vi "类型2自动测试.vi"() -> ()   [LabVIEW 2010]
uses:
  全局量/试验配置信息.vi
panel:
  in  "数组_选择":bool[](array[boolean])
  in  "记录跳变次数":i32
  in  "变化量":dbl
  in  "当前波动值":dbl
  in  "最近一次跳变防线值":i32
  in  "发送值状态":i32
  in  "反馈值":i32
  in  "发送值":dbl
  out "合格？":bool[][](array[boolean])
  in  "跳变值 2":dbl[](array[numeric])
  in  "跳变值 1":dbl[](array[numeric])
  in  "误差":dbl[][](array[numeric])
  out "EVENT_KEY":string
  out "bRece":bool
  out "bSend":bool
  out "bStop":bool
  out "第几组":i32
  # "SEND_RISE = 1,//递增\n\tSEND_SUB = 2,//递减\n\tSEND_OVER = 3//发送完毕"
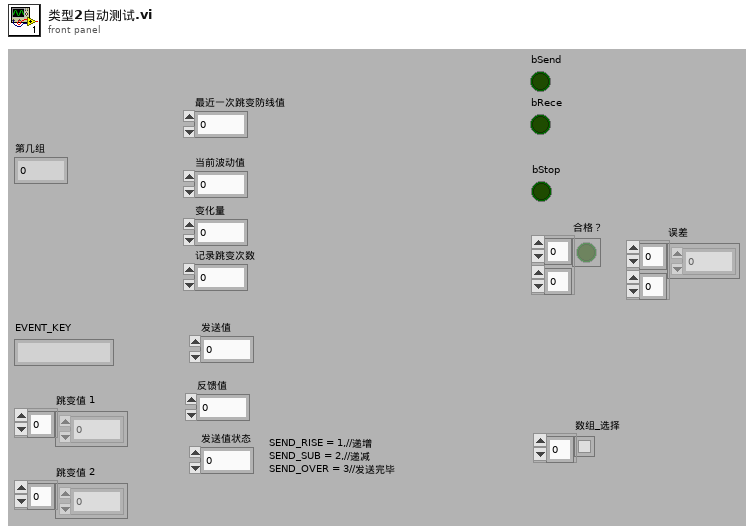
[diagram p1: front panel]
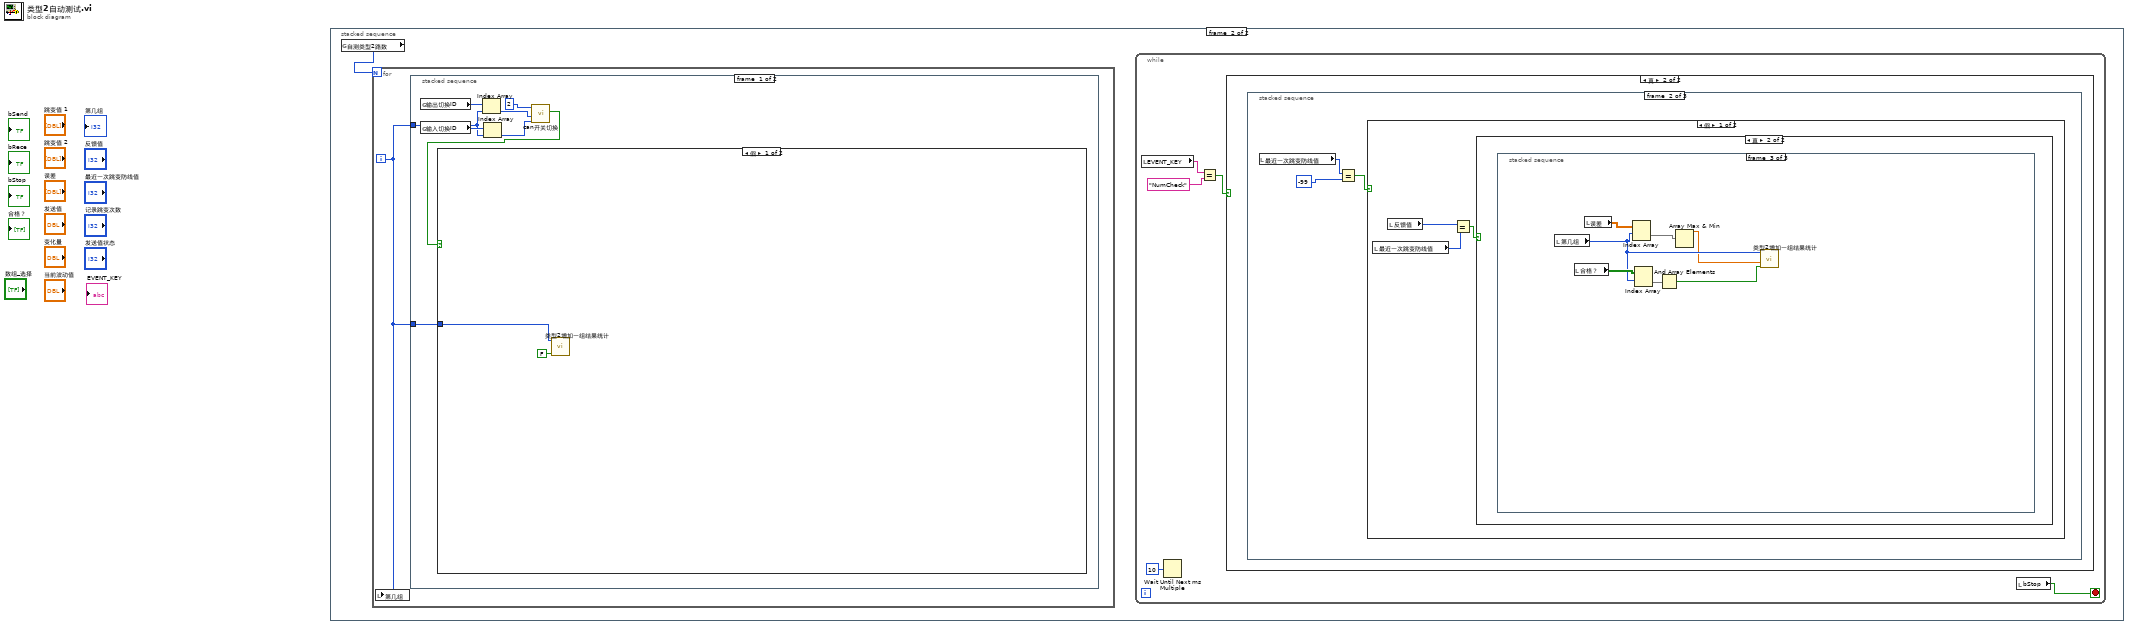
[diagram p0: block diagram]
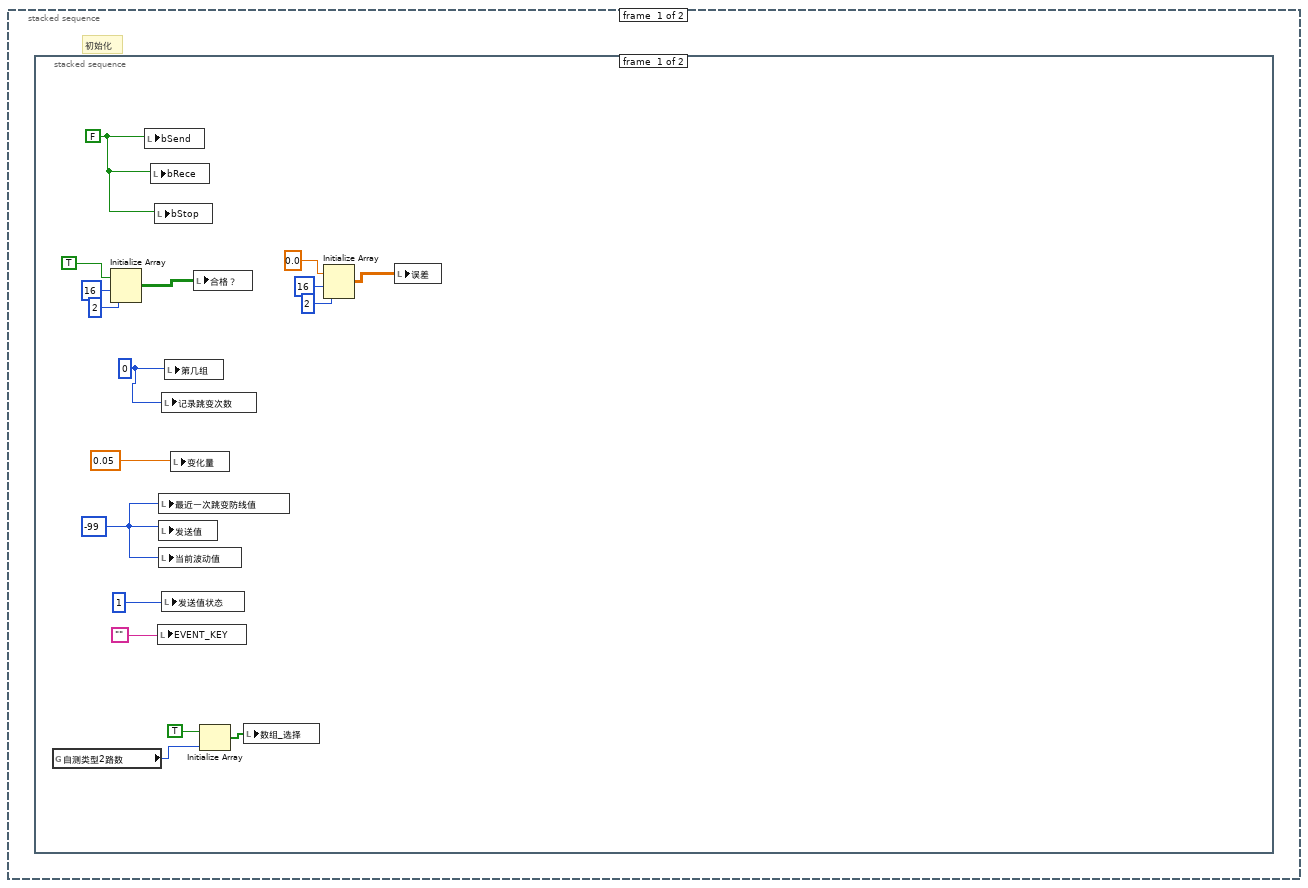
[diagram p2: hidden frame]
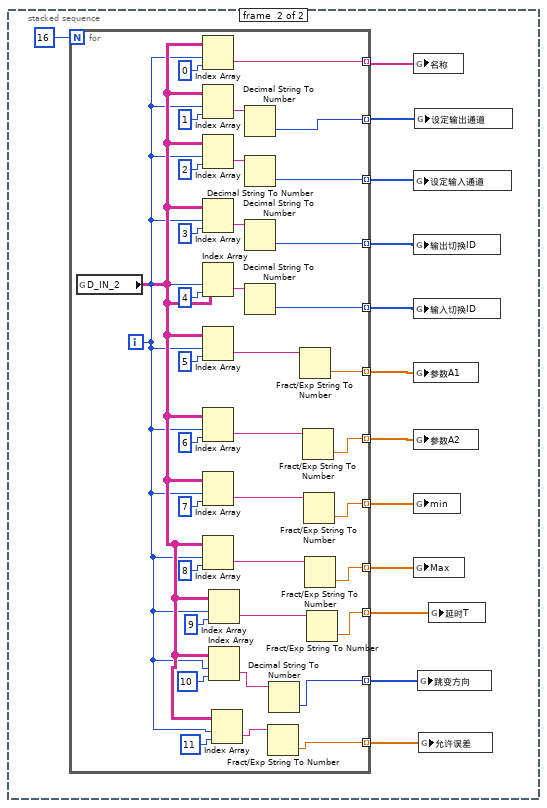
[diagram p3: hidden frame]
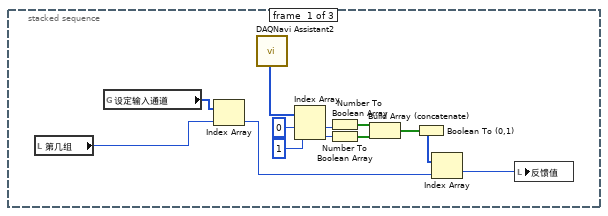
[diagram p5: hidden frame]
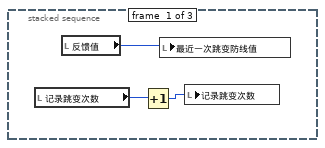
[diagram p7: hidden frame]
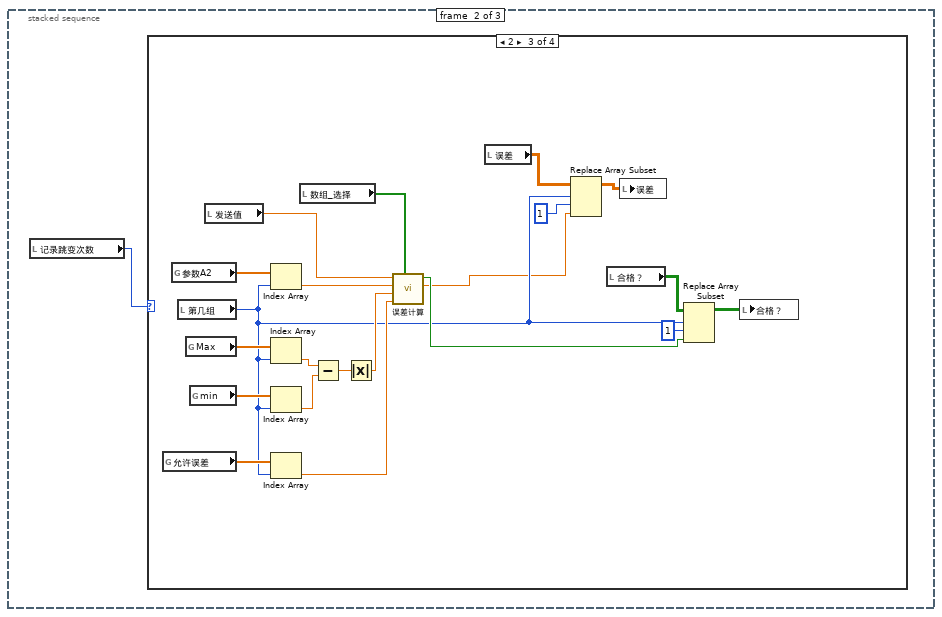
[diagram p8: hidden frame]
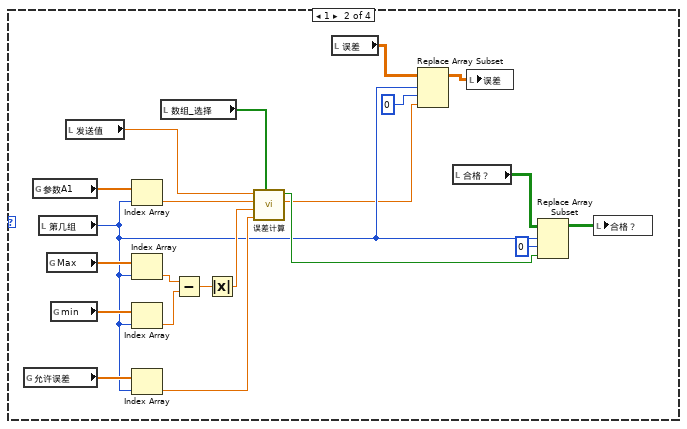
[diagram p10: hidden frame]
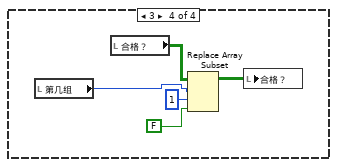
[diagram p11: hidden frame]
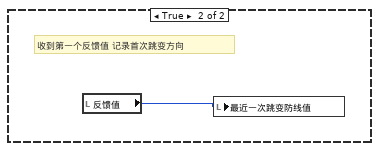
[diagram p12: hidden frame]
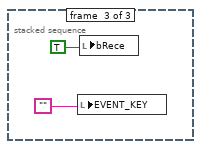
[diagram p13: hidden frame]
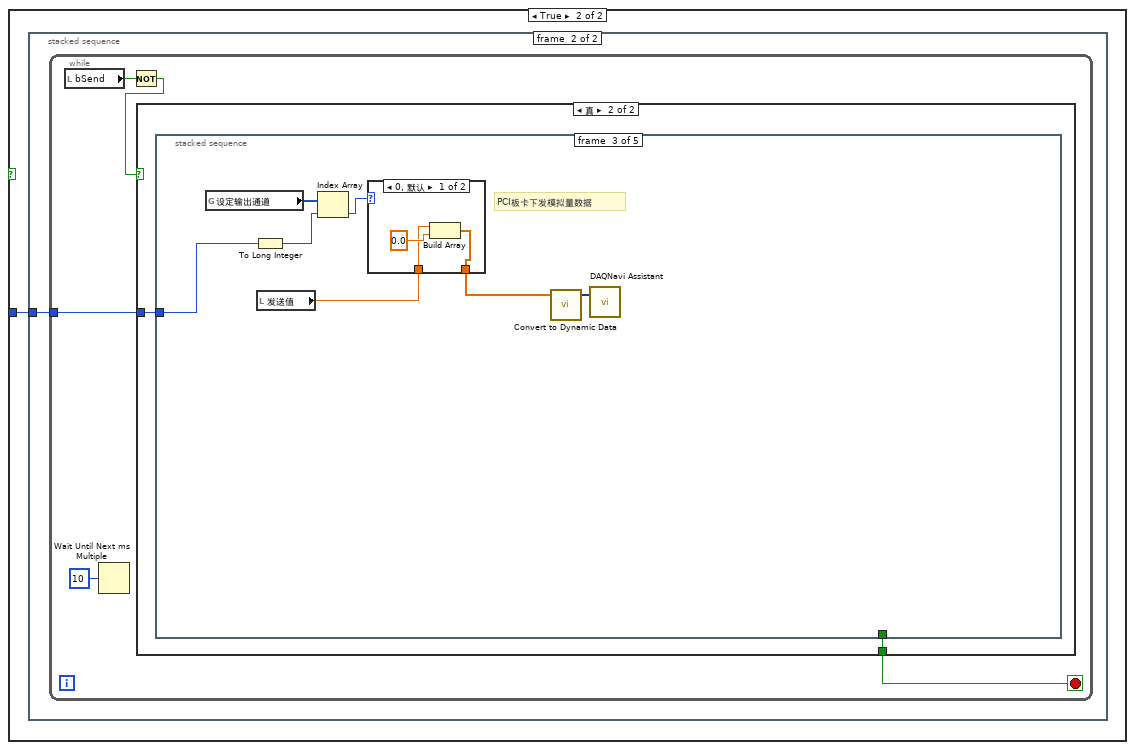
[diagram p14: hidden frame]
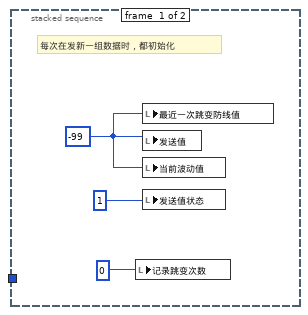
[diagram p15: hidden frame]
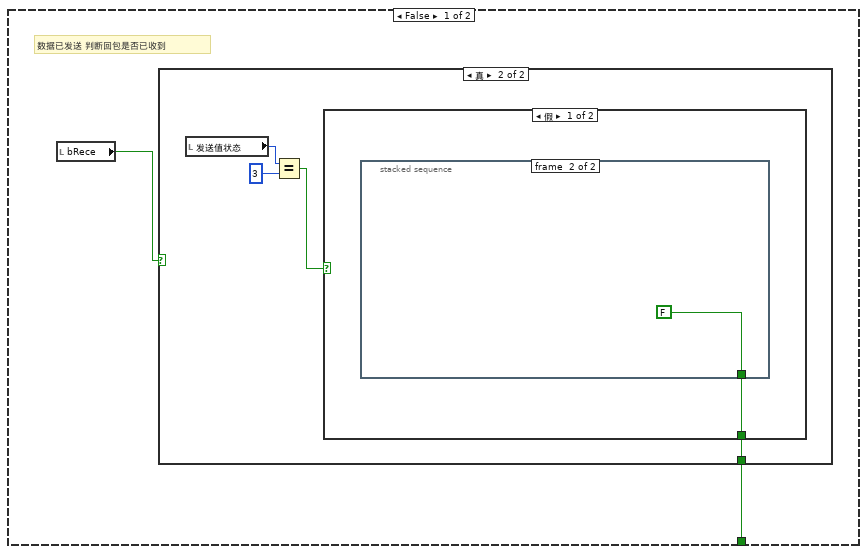
[diagram p16: hidden frame]
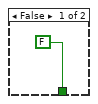
[diagram p17: hidden frame]
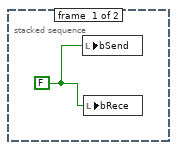
[diagram p18: hidden frame]
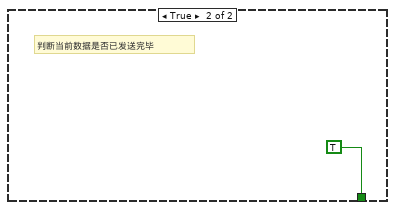
[diagram p19: hidden frame]
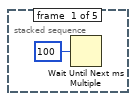
[diagram p20: hidden frame]
diagram:
  n1 = stacked-sequence {
    frame #0 {
      # "初始化"
      n2 = stacked-sequence {
        frame #0 {
          w10 = -99
          w11 = 0
          w17 = FALSE
          n3 = global read "试验配置信息.vi" "自测类型2路数"() -> (w5:i32)
          n4 = Initialize Array(TRUE, 16 ("维数大小"), 2 ("维数大小")) -> (w14:bool[][])
          n5 = local write "bSend"(w17) -> ()
          n6 = local write "bRece"(w17) -> ()
          n7 = local write "bStop"(w17) -> ()
          n8 = local write "EVENT_KEY"("") -> ()
          n9 = local write "最近一次跳变防线值"(w10) -> ()
          n10 = local write "发送值"(w10) -> ()
          n11 = local write "当前波动值"(w10) -> ()
          n12 = local write "记录跳变次数"(w11) -> ()
          n13 = local write "发送值状态"(1) -> ()
          n14 = local write "第几组"(w11) -> ()
          n15 = local write "变化量"(0.05) -> ()
          n16 = local write "合格？"(w14) -> ()
          n17 = Initialize Array(TRUE, w5) -> (w7:bool[])
          n18 = local write "数组_选择"(w7) -> ()
          n19 = Initialize Array(0.0, 16 ("维数大小"), 2 ("维数大小")) -> (w2:dbl[][])
          n20 = local write "误差"(w2) -> ()
        }
        frame #1 {
          n21 = for {
            N: 16 ("维数大小") -> [_]
            tunnel: [w66] -> w24 mode=indexing
            tunnel: [w62] -> w23 mode=indexing
            tunnel: [w60] -> w22 mode=indexing
            tunnel: [w57] -> w21 mode=indexing
            tunnel: [w54] -> w20 mode=indexing
            tunnel: [w51] -> w26 mode=indexing
            tunnel: [w48] -> w27 mode=indexing
            tunnel: [w45] -> w28 mode=indexing
            tunnel: [w42] -> w29 mode=indexing
            tunnel: [w39] -> w30 mode=indexing
            tunnel: [w32] -> w19 mode=indexing
            tunnel: [w31] -> w18 mode=indexing
            i -> [w33]
            n22 = global read "试验配置信息.vi" "D_IN_2"() -> (w34:string[][])
            n23 = Index Array(array=w34, index (row)=w33, index (col)=0 ("禁用的索引 (列)")) -> (element=w66:string)
            n24 = Index Array(array=w34, index (row)=w33, index (col)=1 ("禁用的索引 (列)")) -> (element=w59:string)
            n25 = Index Array(array=w34, index (row)=w33, index (col)=2 ("禁用的索引 (列)")) -> (element=w56:string)
            n26 = Index Array(array=w34, index (row)=w33, index (col)=3 ("禁用的索引 (列)")) -> (element=w52:string)
            n27 = Index Array(array=w34, index (row)=w33, index (col)=4 ("禁用的索引 (列)")) -> (element=w50:string)
            n28 = Index Array(array=w34, index (row)=w33, index (col)=5 ("禁用的索引 (列)")) -> (element=w47:string)
            n29 = Index Array(array=w34, index (row)=w33, index (col)=6 ("禁用的索引 (列)")) -> (element=w43:string)
            n30 = Index Array(array=w34, index (row)=w33, index (col)=7 ("禁用的索引 (列)")) -> (element=w63:string)
            n31 = Index Array(array=w34, index (row)=w33, index (col)=8 ("禁用的索引 (列)")) -> (element=w61:string)
            n32 = Index Array(array=w34, index (row)=w33, index (col)=9 ("禁用的索引 (列)")) -> (element=w40:string)
            n33 = Index Array(array=w34, index (row)=w33, index (col)=10 ("禁用的索引 (列)")) -> (element=w35:string)
            n34 = Index Array(array=w34, index (row)=w33, index (col)=11 ("禁用的索引 (列)")) -> (element=w36:string)
            n35 = Decimal String To Number(string=w59) -> (number=w57:i32)  [unwired: 2 in, 1 out]
            n36 = Decimal String To Number(string=w56) -> (number=w54:i32)  [unwired: 2 in, 1 out]
            n37 = Decimal String To Number(string=w52) -> (number=w51:i32)  [unwired: 2 in, 1 out]
            n38 = Decimal String To Number(string=w50) -> (number=w48:i32)  [unwired: 2 in, 1 out]
            n39 = Fract/Exp String To Number(string=w36) -> (number=w31:dbl)  [unwired: 3 in, 1 out]
            n40 = Decimal String To Number(string=w35) -> (number=w32:i32)  [unwired: 2 in, 1 out]
            n41 = Fract/Exp String To Number(string=w47) -> (number=w45:dbl)  [unwired: 3 in, 1 out]
            n42 = Fract/Exp String To Number(string=w43) -> (number=w42:dbl)  [unwired: 3 in, 1 out]
            n43 = Fract/Exp String To Number(string=w63) -> (number=w62:dbl)  [unwired: 3 in, 1 out]
            n44 = Fract/Exp String To Number(string=w61) -> (number=w60:dbl)  [unwired: 3 in, 1 out]
            n45 = Fract/Exp String To Number(string=w40) -> (number=w39:dbl)  [unwired: 3 in, 1 out]
          }
          n46 = global write "试验配置信息.vi" "名称"(w24) -> ()
          n47 = global write "试验配置信息.vi" "设定输入通道"(w20) -> ()
          n48 = global write "试验配置信息.vi" "输出切换ID"(w26) -> ()
          n49 = global write "试验配置信息.vi" "输入切换ID"(w27) -> ()
          n50 = global write "试验配置信息.vi" "参数A1"(w28) -> ()
          n51 = global write "试验配置信息.vi" "参数A2"(w29) -> ()
          n52 = global write "试验配置信息.vi" "min"(w23) -> ()
          n53 = global write "试验配置信息.vi" "Max"(w22) -> ()
          n54 = global write "试验配置信息.vi" "设定输出通道"(w21) -> ()
          n55 = global write "试验配置信息.vi" "跳变方向"(w19) -> ()
          n56 = global write "试验配置信息.vi" "允许误差"(w18) -> ()
          n57 = global write "试验配置信息.vi" "延时T"(w30) -> ()
        }
      }
    }
    frame #1 {
      n58 = global read "试验配置信息.vi" "自测类型2路数"() -> (w68:i32)
      n59 = for {
        N: w68 -> [_]
        i -> [w154]
        n60 = local write "第几组"(w154) -> ()
        n61 = stacked-sequence {
          tunnel: w154 -> [w157 _]
          tunnel: w154 -> [w155 _]
          frame #0 {
            n62 = global read "试验配置信息.vi" "输出切换ID"() -> (w159:i32[])
            n63 = global read "试验配置信息.vi" "输入切换ID"() -> (w160:i32[])
            n64 = Index Array(array=w159, index=w157) -> (element=w158:i32)
            n65 = Index Array(array=w160, index=w157) -> (element=w161:i32)
            n66 = call "can开关切换.vi"("输入切换ID"=w161, "输出切换ID"=w158, "函数类型"=2) -> ("成功？"=w156:bool)  [unwired: 7 in]
            n67 = case shown="假" w156 {
              tunnel: w155 -> [w164 w165]
              frame False {
                n68 = call "类型2增加一组结果统计.vi"("合格"=FALSE, "第几组"=w164) -> ()  [unwired: 10 in]
              }
              frame True {
                n69 = stacked-sequence {
                  tunnel: w165 -> [_ w169]
                  frame #0 {
                    w168 = -99
                    # "每次在发新一组数据时，都初始化"
                    n70 = local write "记录跳变次数"(0) -> ()
                    n71 = local write "最近一次跳变防线值"(w168) -> ()
                    n72 = local write "发送值"(w168) -> ()
                    n73 = local write "当前波动值"(w168) -> ()
                    n74 = local write "发送值状态"(1) -> ()
                  }
                  frame #1 {
                    n75 = while {
                      tunnel: w169 -> [w172]
                      stop <- w171 stop-if-true
                      n76 = local read "bSend"() -> (w174:bool)
                      n77 = Wait Until Next ms Multiple(millisecond multiple=u32 10 ("毫秒倍数")) -> ()  [unwired: 1 out]
                      n78 = Not(x=w174) -> (.not. x?=w173:bool)
                      n79 = case shown="真" w173 {
                        tunnel: w172 -> [_ w187]
                        tunnel: [w175 w186] -> w171
                        frame False {
                          # "数据已发送 判断回包是否已收到"
                          n80 = local read "bRece"() -> (w176:bool)
                          n81 = case shown="真" w176 {
                            tunnel: [FALSE w178] -> w175
                            frame False {
                            }
                            frame True {
                              n82 = local read "发送值状态"() -> (w181:i32)
                              n83 = Equal?(x=w181, y=3) -> (x = y?=w179:bool)
                              n84 = case shown="假" w179 {
                                tunnel: [w182 TRUE] -> w178
                                frame False {
                                n85 = stacked-sequence {
                                tunnel: [_ FALSE] -> w182
                                frame #0 {
                                w183 = FALSE
                                n86 = local write "bSend"(w183) -> ()
                                n87 = local write "bRece"(w183) -> ()
                                }
                                frame #1 {
                                }
                                }
                                }
                                frame True {
                                # "判断当前数据是否已发送完毕"
                                }
                              }
                            }
                          }
                        }
                        frame True {
                          n88 = stacked-sequence {
                            tunnel: w187 -> [_ _ w216 _ _]
                            tunnel: [_ _ _ _ FALSE] -> w186
                            frame #0 {
                              n89 = Wait Until Next ms Multiple(millisecond multiple=u32 100 ("毫秒倍数")) -> ()  [unwired: 1 out]
                            }
                            frame #1 {
                              n90 = local read "发送值"() -> (w191:dbl)
                              n91 = Equal?(x=w191, y=-99.0) -> (x = y?=w189:bool)
                              n92 = case shown="假" w189 {
                                frame False {
                                n93 = local read "发送值状态"() -> (w192:i32)
                                n94 = case shown="1, 默认" w192 {
                                frame 1, Default {
                                # "当前状态是递增"
                                n95 = stacked-sequence {
                                frame #0 {
                                n96 = local read "发送值"() -> (w195:dbl)
                                n97 = local read "变化量"() -> (w194:dbl)
                                n98 = Add(x=w195, y=w194) -> (x+y=w193:dbl)
                                n99 = local write "发送值"(w193) -> ()
                                }
                                frame #1 {
                                n100 = local read "第几组"() -> (w199:i32)
                                n101 = global read "试验配置信息.vi" "Max"() -> (w200:dbl[])
                                n102 = local read "发送值"() -> (w198:dbl)
                                n103 = Index Array(array=w200, index=w199) -> (element=w196:dbl)
                                n104 = Greater Or Equal?(x=w198, y=w196) -> (x >= y?=w197:bool)
                                n105 = case shown="真" w197 {
                                tunnel: w196 -> [_ w202]
                                frame False {
                                }
                                frame True {
                                # "超过最大值时\n将状态改为递减状态"
                                n106 = local write "发送值"(w202) -> ()
                                n107 = local write "发送值状态"(2 ("发送值状态")) -> ()
                                }
                                }
                                }
                                }
                                }
                                frame 2 {
                                # "当前状态为递减状态"
                                n108 = stacked-sequence {
                                frame #0 {
                                n109 = local read "发送值"() -> (w205:dbl)
                                n110 = local read "变化量"() -> (w204:dbl)
                                n111 = Subtract(x=w205, y=w204) -> (x-y=w203:dbl)
                                n112 = local write "发送值"(w203) -> ()
                                }
                                frame #1 {
                                n113 = local read "第几组"() -> (w209:i32)
                                n114 = global read "试验配置信息.vi" "min"() -> (w210:dbl[])
                                n115 = local read "发送值"() -> (w208:dbl)
                                n116 = Index Array(array=w210, index=w209) -> (element=w206:dbl)
                                n117 = Less Or Equal?(x=w208, y=w206) -> (x <= y?=w207:bool)
                                n118 = case shown="真" w207 {
                                tunnel: w206 -> [_ w212]
                                frame False {
                                }
                                frame True {
                                # "递减到最小值时 代表发送了一个周期"
                                n119 = local write "发送值"(w212) -> ()
                                n120 = local write "发送值状态"(3 ("发送值状态")) -> ()
                                }
                                }
                                }
                                }
                                }
                                }
                                }
                                frame True {
                                # "默认值 证明为发送的第一条数据\n从最小值开始"
                                n121 = local read "第几组"() -> (w213:i32)
                                n122 = global read "试验配置信息.vi" "min"() -> (w215:dbl[])
                                n123 = Index Array(array=w215, index=w213) -> (element=w214:dbl)
                                n124 = local write "发送值"(w214) -> ()
                                }
                              }
                            }
                            frame #2 {
                              # "PCI板卡下发模拟量数据"
                              n125 = global read "试验配置信息.vi" "设定输出通道"() -> (w222:i32[])
                              n126 = To Long Integer(number=w216) -> (32bit integer=w221:i32)
                              n127 = local read "发送值"() -> (w217:dbl)
                              n128 = Index Array(array=w222, index=w221) -> (element=w218:i32)
                              n129 = case shown="0, 默认" w218 {
                                tunnel: [w225 w228] -> w219
                                tunnel: w217 -> [w223 w226]
                                frame 0, Default {
                                n130 = Build Array(w223, 0.0) -> (w225:dbl[])
                                }
                                frame 1 {
                                n131 = Build Array(0.0, w226) -> (w228:dbl[])
                                }
                              }
                              n132 = call "Convert to Dynamic Data"("Array"=w219) -> ("Dynamic Data Type"=w220:dynamicdata)  [unwired: 3 out]
                              n133 = call "DAQNavi Assistant"("data in(DDT)"=w220) -> ()  [unwired: 2 in, 17 out]
                            }
                            frame #3 {
                              n134 = local write "EVENT_KEY"("NumCheck") -> ()
                            }
                            frame #4 {
                              n135 = local write "bSend"(TRUE) -> ()
                            }
                          }
                        }
                      }
                    }
                  }
                }
              }
            }
          }
          frame #1 {
            n136 = local read "第几组"() -> (w233:i32)
            n137 = global read "试验配置信息.vi" "自测类型2路数"() -> (w235:i32)
            n138 = Decrement(x=w235) -> (x-1=w234:i32)
            n139 = Equal?(x=w234, y=w233) -> (x = y?=w232:bool)
            n140 = local write "bStop"(w232) -> ()
          }
        }
      }
      n141 = while {
        stop <- w73 stop-if-true
        n142 = local read "EVENT_KEY"() -> (w71:string)
        n143 = Wait Until Next ms Multiple(millisecond multiple=u32 10 ("毫秒倍数")) -> ()  [unwired: 1 out]
        n144 = Equal?(x=w71, y="NumCheck") -> (x = y?=w69:bool)
        n145 = case shown="真" w69 {
          frame False {
          }
          frame True {
            n146 = stacked-sequence {
              frame #0 {
                n147 = local read "第几组"() -> (w76:i32)
                n148 = global read "试验配置信息.vi" "设定输入通道"() -> (w77:i32[])
                n149 = Index Array(array=w77, index=w76) -> (element=w75:i32)
                n150 = call "DAQNavi Assistant2"() -> ("dataOut(U8Array)"=w78:u8[])  [unwired: 2 in, 17 out]
                n151 = Index Array(array=w78, index #1=0 ("索引"), index #2=1 ("索引")) -> (element #1=w83:u8, element #2=w84:u8)
                n152 = Number To Boolean Array(number=w83) -> (Boolean array=w79:bool[])
                n153 = Number To Boolean Array(number=w84) -> (Boolean array=w80:bool[])
                n154 = Build Array (concatenate)(w79, w80) -> (w85:bool[])
                n155 = Boolean To (0,1) ("布尔值至(0,1)转换")(Boolean=w85) -> (0, 1=w86:i16[])
                n156 = Index Array(array=w86, index=w75) -> (element=w74:i16)
                n157 = local write "反馈值"(w74) -> ()
              }
              frame #1 {
                n158 = local read "最近一次跳变防线值"() -> (w89:i32)
                n159 = Equal?(x=w89, y=-99) -> (x = y?=w87:bool)
                n160 = case shown="假" w87 {
                  frame False {
                    n161 = local read "最近一次跳变防线值"() -> (w90:i32)
                    n162 = local read "反馈值"() -> (w92:i32)
                    n163 = Equal?(x=w92, y=w90) -> (x = y?=w91:bool)
                    n164 = case shown="真" w91 {
                      frame False {
                      }
                      frame True {
                        n165 = stacked-sequence {
                          frame #0 {
                            n166 = local read "记录跳变次数"() -> (w94:i32)
                            n167 = local read "反馈值"() -> (w95:i32)
                            n168 = Increment(x=w94) -> (x+1=w93:i32)
                            n169 = local write "最近一次跳变防线值"(w95) -> ()
                            n170 = local write "记录跳变次数"(w93) -> ()
                          }
                          frame #1 {
                            n171 = local read "记录跳变次数"() -> (w96:i32)
                            n172 = case shown="2" w96 {
                              frame 0, Default {
                              }
                              frame 1 {
                                n173 = global read "试验配置信息.vi" "允许误差"() -> (w114:dbl[])
                                n174 = global read "试验配置信息.vi" "参数A1"() -> (w117:dbl[])
                                n175 = local read "第几组"() -> (w98:i32)
                                n176 = global read "试验配置信息.vi" "Max"() -> (w116:dbl[])
                                n177 = global read "试验配置信息.vi" "min"() -> (w115:dbl[])
                                n178 = local read "发送值"() -> (w113:dbl)
                                n179 = Index Array(array=w117, index=w98) -> (element=w112:dbl)
                                n180 = Index Array(array=w116, index=w98) -> (element=w111:dbl)
                                n181 = Index Array(array=w115, index=w98) -> (element=w110:dbl)
                                n182 = Index Array(array=w114, index=w98) -> (element=w107:dbl)
                                n183 = local read "数组_选择"() -> (w106:bool[])
                                n184 = Subtract(x=w111, y=w110) -> (x-y=w109:dbl)
                                n185 = Absolute Value(x=w109) -> (abs(x)=w108:dbl)
                                n186 = call "误差计算.vi"("选择?"=w106, "允许误差"=w107, "模拟量量程范围"=w108, "设定值_1"=w112, "反馈值_1"=w113) -> ("误差_1"=w97:dbl, "合格_1?"=w102:bool)  [unwired: 4 in, 1 out]
                                n187 = local read "误差"() -> (w101:dbl[][])
                                n188 = Replace Array Subset(array=w101, new element=w97, index (row)=w98, index (col)=0 ("禁用的索引 (列)")) -> (w100:dbl[][])
                                n189 = local read "合格？"() -> (w105:bool[][])
                                n190 = local write "误差"(w100) -> ()
                                n191 = Replace Array Subset(array=w105, new element=w102, index (row)=w98, index (col)=0 ("禁用的索引 (列)")) -> (w104:bool[][])
                                n192 = local write "合格？"(w104) -> ()
                              }
                              frame 2 {
                                n193 = global read "试验配置信息.vi" "允许误差"() -> (w135:dbl[])
                                n194 = global read "试验配置信息.vi" "参数A2"() -> (w138:dbl[])
                                n195 = local read "第几组"() -> (w120:i32)
                                n196 = global read "试验配置信息.vi" "Max"() -> (w137:dbl[])
                                n197 = global read "试验配置信息.vi" "min"() -> (w136:dbl[])
                                n198 = local read "发送值"() -> (w134:dbl)
                                n199 = Index Array(array=w138, index=w120) -> (element=w133:dbl)
                                n200 = Index Array(array=w137, index=w120) -> (element=w132:dbl)
                                n201 = Index Array(array=w136, index=w120) -> (element=w131:dbl)
                                n202 = Index Array(array=w135, index=w120) -> (element=w128:dbl)
                                n203 = local read "数组_选择"() -> (w127:bool[])
                                n204 = Subtract(x=w132, y=w131) -> (x-y=w130:dbl)
                                n205 = Absolute Value(x=w130) -> (abs(x)=w129:dbl)
                                n206 = call "误差计算.vi"("选择?"=w127, "允许误差"=w128, "模拟量量程范围"=w129, "设定值_1"=w133, "反馈值_1"=w134) -> ("误差_1"=w118:dbl, "合格_1?"=w123:bool)  [unwired: 4 in, 1 out]
                                n207 = local read "误差"() -> (w122:dbl[][])
                                n208 = Replace Array Subset(array=w122, new element=w118, index (row)=w120, index (col)=1 ("禁用的索引 (列)")) -> (w121:dbl[][])
                                n209 = local read "合格？"() -> (w126:bool[][])
                                n210 = local write "误差"(w121) -> ()
                                n211 = Replace Array Subset(array=w126, new element=w123, index (row)=w120, index (col)=1 ("禁用的索引 (列)")) -> (w125:bool[][])
                                n212 = local write "合格？"(w125) -> ()
                              }
                              frame 3 {
                                n213 = local read "第几组"() -> (w140:i32)
                                n214 = local read "合格？"() -> (w143:bool[][])
                                n215 = Replace Array Subset(array=w143, new element=FALSE, index (row)=w140, index (col)=1 ("禁用的索引 (列)")) -> (w142:bool[][])
                                n216 = local write "合格？"(w142) -> ()
                              }
                            }
                          }
                          frame #2 {
                            n217 = local read "第几组"() -> (w146:i32)
                            n218 = local read "合格？"() -> (w149:bool[][])
                            n219 = local read "误差"() -> (w150:dbl[][])
                            n220 = Index Array(array=w150, index (row)=w146) -> (element=w147:dbl[])  [unwired: 1 in]
                            n221 = Index Array(array=w149, index (row)=w146) -> (element=w148:bool[])  [unwired: 1 in]
                            n222 = And Array Elements(Boolean array=w148) -> (logical AND=w144:bool)
                            n223 = Array Max & Min(array=w147) -> (max value=w145:dbl)  [unwired: 3 out]
                            n224 = call "类型2增加一组结果统计.vi"("合格"=w144, "最大误差"=w145, "第几组"=w146) -> ()  [unwired: 9 in]
                          }
                        }
                      }
                    }
                  }
                  frame True {
                    # "收到第一个反馈值 记录首次跳变方向"
                    n225 = local read "反馈值"() -> (w151:i32)
                    n226 = local write "最近一次跳变防线值"(w151) -> ()
                  }
                }
              }
              frame #2 {
                n227 = local write "EVENT_KEY"("") -> ()
                n228 = local write "bRece"(TRUE) -> ()
              }
            }
          }
        }
        n229 = local read "bStop"() -> (w73:bool)
      }
    }
  }
